vi "블록 다이어그램.vi"() -> ()   [LabVIEW 2010]
uses:
  <vilib>/NXT/Block Support/NXT_InputPort.ctl
  <vilib>/NXT/Subs/MotorOutput.ctl
  <vilib>/NXT/Dual Mode Library/Motors/MotorOn.vi
panel:
  in  "Port (Port 3) 2":T1=2 items=["Port 1", "Port 2", "Port 3", "Port 4"]
  in  "Port (Port 3)":T1=2 items=["Port 1", "Port 2", "Port 3", "Port 4"]
  in  "Power (75)":i32=75
  in  "stop":bool
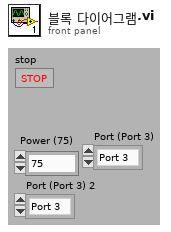
[diagram p1: front panel]
types:
  T1 = typedef "NXT_InputPort.ctl" = u8
  T2 = typedef "MotorOutput.ctl" = u8
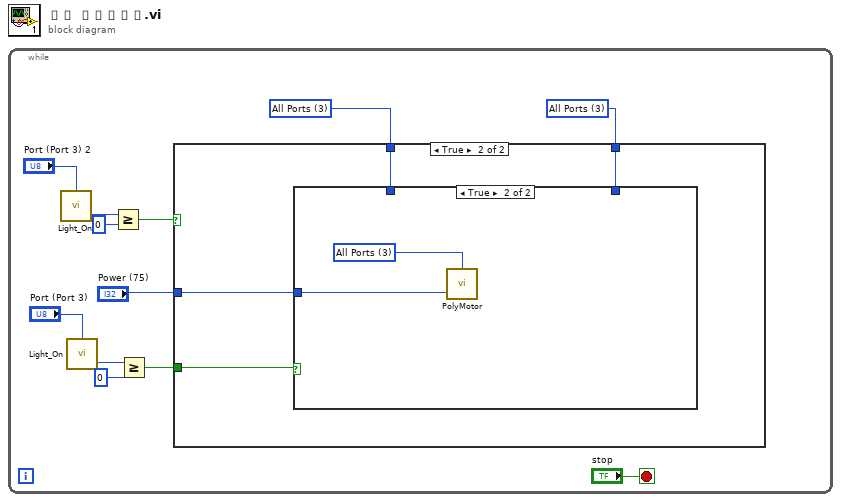
[diagram p0: block diagram]
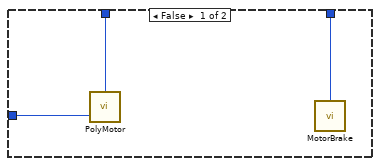
[diagram p3: hidden frame]
diagram:
  n1 = while {
    stop <- "stop" stop-if-true
    w10 = T2 3 items=["Port A", "Port B", "Port C", "All Ports"] ("Port (All Ports)")
    w11 = T2 3 items=["Port A", "Port B", "Port C", "All Ports"] ("Output Port (All Ports)")
    n2 = call <vilib>:"Light_On.vi"("Port (Port 3)"="Port (Port 3) 2") -> ("Scaled Value"=w6:i16)  [unwired: 2 in, 1 out]
    n3 = call <vilib>:"Light_On.vi"("Port (Port 3)"="Port (Port 3)") -> ("Scaled Value"=w5:i16)  [unwired: 2 in, 1 out]
    n4 = Greater Or Equal?(x=w6, y=i16 0) -> (x >= y?=w2:bool)
    n5 = Greater Or Equal?(x=w5, y=i16 0) -> (x >= y?=w1:bool)
    n6 = case shown="True" w2 {
      tunnel: w11 -> [_ w16]
      tunnel: w10 -> [_ w15]
      tunnel: "Power (75)" -> [_ w14]
      tunnel: w1 -> [_ w13]
      frame False {
      }
      frame True {
        n7 = case shown="True" w13 {
          tunnel: w16 -> [w19 _]
          tunnel: w15 -> [w18 _]
          tunnel: w14 -> [w17 w20]
          frame False {
            n8 = call-poly <vilib>:"PolyMotor.vi"("Power (75)"=w17, "Output Port (All Ports)"=w19) -> ()  [unwired: 2 in, 1 out]
            n9 = call <vilib>:"MotorBrake.vi"("Port (All Ports)"=w18) -> ()  [unwired: 3 in, 1 out]
          }
          frame True {
            w21 = T2 3 items=["Port A", "Port B", "Port C", "All Ports"] ("Output Port (All Ports)")
            n10 = call-poly <vilib>:"PolyMotor.vi"("Power (75)"=w20, "Output Port (All Ports)"=w21) -> ()  [unwired: 2 in, 1 out]
          }
        }
      }
    }
  }
